vi "Serialize.vi"(8 "error in (no error)":errorcluster, 11 "VIP Install in":refnum<class "VIP Install.lvclass">) -> (0 "error out":errorcluster, 2 "Text":string)   [LabVIEW 2014, in "VIP Install.lvclass"]
uses:
  VIP Install.lvclass
  VIP Install - STYP.ctl
  VIP Install.lvclass/VIP Install.ctl
  Read LV Version.vi
  Read VIP Name.vi
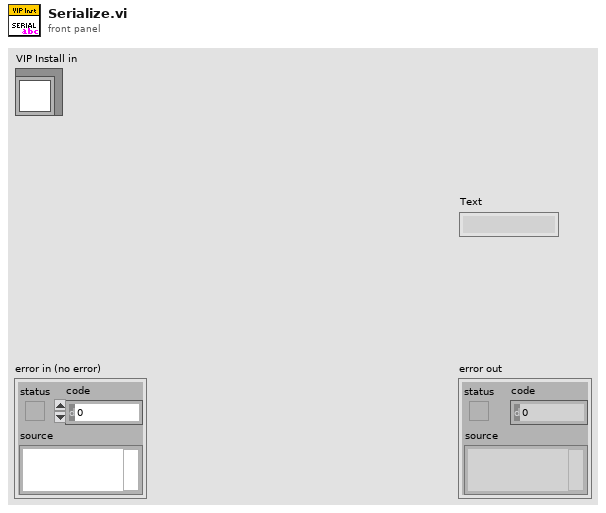
[diagram p1: front panel]
types:
  T1 = typedef "VIP Install - STYP.ctl" = cluster{"VIP Name":string, "LabVIEW Version":string}
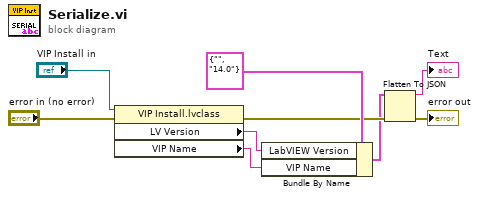
[diagram p0: block diagram]
diagram:
  n1 = property class="VIP Install.lvclass"(reference="VIP Install in", error in="error in (no error)") -> (error out=w4:errorcluster, "LV Version"=w6:string, "VIP Name"=w5:string)  [unwired: 1 out]
  n2 = Bundle By Name(cluster=T1 {"VIP Name"="", "LabVIEW Version"="14.0"} ("VIP Install"), "LabVIEW Version"=w6, "VIP Name"=w5) -> (w2:T1)
  n3 = Flatten To JSON(anything=w2, error in (no error)=w4) -> (JSON string=→"Text":string, 11:→"error out":errorcluster)  [unwired: 1 in]
